vi "Status Dialog.vi"(11 "queue in":refnum<queue>) -> ()   [LabVIEW 2026, in "NIVS_CDEW_MetaDataObj.lvclass"]
uses:
  NIVS_CDEW_MetaDataObj.lvclass
panel:
  in  "?":string="Starting Custom Device projects creation. This could take several minutes."
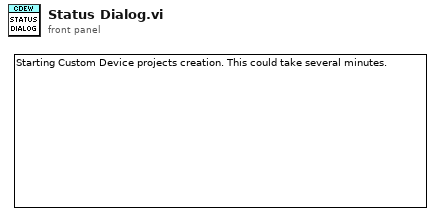
[diagram p1: front panel]
types:
  T1 = enum16{"Create CD Root Folder", "Copy Compiled Settings", "Generate Custom Device DLL from XML", "Calculate Page Properties", "Create Configuration Project", "Create Engine Project", "Create Custom Device Engine Project", "Create System Explorer Project", "Create Test Hooks Project", "Relink and Clean Up VIs", "Build PPLs", "Copy Custom Device DLL to Public Documents", "Open Projects", "Shutdown"}
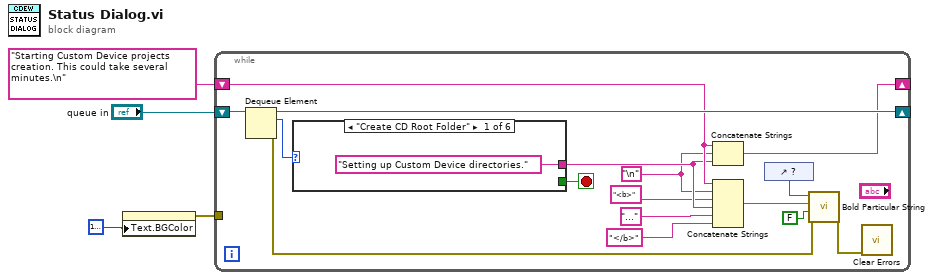
[diagram p0: block diagram]
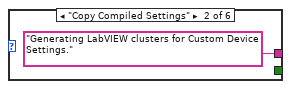
[diagram p2: hidden frame]
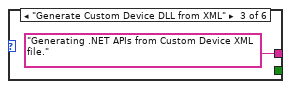
[diagram p3: hidden frame]
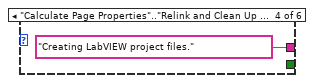
[diagram p4: hidden frame]
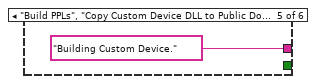
[diagram p5: hidden frame]
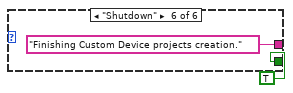
[diagram p6: hidden frame]
diagram:
  n1 = property class="Str"("Text.BGColor"=u32 16777226 ("Text.Text Colors:BG Color")) -> (error out=w1:errorcluster)  [unwired: 2 in, 1 out]
  n2 = while {
    shift-right: [w19] -> _
    shift-left: "queue in" -> [w20]
    shift-right: [w17] -> _
    shift-left: "Starting Custom Device projects creation. This could take several minutes.\n" -> [w15]
    tunnel: w1 -> [_]
    stop <- w16 stop-if-true
    w5 = "\n"
    n3 = Dequeue Element(queue=w20) -> (queue out=w19:refnum<queue>, element=w18:T1, error out=w7:errorcluster)  [unwired: 2 in, 1 out]
    n4 = case shown="\"Create CD Root Folder\"" w18 {
      tunnel: ["Setting up Custom Device directories." "Generating LabVIEW clusters for Custom Device Settings." "Generating .NET APIs from Custom Device XML file." "Creating LabVIEW project files." "Building Custom Device." "Finishing Custom Device projects creation."] -> w14
      tunnel: [_ _ _ _ _ TRUE] -> w16
      frame "Create CD Root Folder" {
      }
      frame "Copy Compiled Settings" {
      }
      frame "Generate Custom Device DLL from XML" {
      }
      frame "Calculate Page Properties".."Relink and Clean Up VIs", "Open Projects" {
      }
      frame "Build PPLs", "Copy Custom Device DLL to Public Documents" {
      }
      frame "Shutdown" {
      }
    }
    n5 = Concatenate Strings(w15, w5, w14) -> (w17:string)
    n6 = Concatenate Strings(w15, w5, "<b>" ("string"), w14, "..." ("string"), "</b>" ("string")) -> (w11:string)
    n7 = control-ref of="?"() -> (w12:refnum<vi>)
    n8 = call <vilib>:"Bold Particular String.vi"("error in (no error)"=w7, "resize string? (TRUE)"=FALSE, "text to display"=w11, "string refnum"=w12) -> ("error out"=w6:errorcluster)  [unwired: 6 in, 1 out]
    n9 = call <vilib>:"Clear Errors.vi"("error in (no error)"=w6) -> ()  [unwired: 5 in, 2 out]
  }
